vi "WriteGroupedDigitalOutputs.vi"(8 "error in (no error)":errorcluster, 10 "data":u32, 11 "TesteractHAL_DigitalIO In":refnum<class "TesteractHAL_DigitalOutput.lvclass">) -> (0 "error out":errorcluster, 3 "TesteractHAL_DigitalIO Out":refnum<class "TesteractHAL_DigitalOutput.lvclass">)   [LabVIEW 2017, in "TesteractHAL_DigitalOutput.lvlib" / "TesteractHAL_DigitalOutput.lvclass"]
doc: "Write a single digital channel where the number represents the bits to set on the digital signal."
uses:
  TesteractHAL_DigitalOutput.lvclass
  Program Files (x86)/Testeract/HWLib/HAL/Device/TesteractHAL_Device.lvlibp/TesteractHAL_Device.lvclass
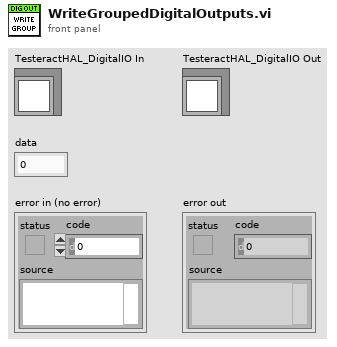
[diagram p1: front panel]
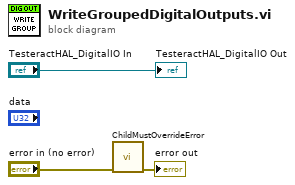
[diagram p0: block diagram]
diagram:
  n1 = call "ChildMustOverrideError.vi"("error in (no error)"="error in (no error)") -> ("error out"=→"error out":errorcluster)  [unwired: 10 in]
  "TesteractHAL_DigitalIO Out" <- "TesteractHAL_DigitalIO In"
